vi "1DTurnMainTester.vi"() -> ()   [LabVIEW 2017]
uses:
  <vilib>/Rock Robotics/WPI/SafetyOutput/WPI_SafetyOutputConfigMenu.ctl
  <vilib>/Rock Robotics/SystemInterfaces/DIO/FPGA_DIOPWMChannel.ctl
  <vilib>/Rock Robotics/SystemInterfaces/DIO/FPGA_DIOChannel.ctl
  <extravilib>/ChannelInstances/Lossy Stream-c(dbl,dbl,dbl,dbl,dbl,dbl)/Write With Abort.vi
  <extravilib>/ChannelInstances/Lossy Stream-c(dbl,dbl,dbl,dbl,dbl,dbl)/Read With Abort.vi
  <extravilib>/ChannelInstances/Lossy Stream-c(dbl,dbl,dbl,dbl,dbl,dbl)/Endpoint.vi
  <extravilib>/ChannelInstances/Lossy Stream-c(dbl,dbl,dbl,dbl,dbl,dbl)/EndpointRead.vi
  <vilib>/Rock Robotics/WPI/RobotDrive/WPI_RobotDriveOpen4MotorWithSPARK.vi
  <vilib>/Rock Robotics/WPI/RobotDrive/WPI_RobotDriveOpen2MotorWithSPARK.vi
  <vilib>/Rock Robotics/WPI/Counter/WPI_CounterDigitalInputToDigitalSource.vi
  <extravilib>/ChannelInstances/Lossy Stream-c(dbl,dbl,dbl,dbl,dbl,dbl)/Instantiate.vi
  <extravilib>/ChannelInstances/Lossy Stream-c(dbl,dbl,dbl,dbl,dbl,dbl)/)Channel.vi
  <resource>/ChannelSupport/_ChannelSupport/WaitIfNeeded.vi
  <vilib>/Rock Robotics/WPI/ThirdParty/Sensors/navX/_Processing Loop/FRIC_navX_Internal_SPI_ProcessingLoop.vi
  <extravilib>/ChannelInstances/Lossy Stream-c(dbl,dbl,dbl,dbl,dbl,dbl).lvlib
panel:
  out "Trackwidth":dbl(graph)=25.77061221384658
  in  "AutoTurnSpeed":dbl=0.7
  in  "ThingToDo":enum16{"TestTurning", "FindTrackwidth"}(ring)
  out "Encoder Position":cluster{"Distance":dbl, "CurrentAngle":dbl}(graph)
  in  "Gains":T1={"Gains"={"FFV"=0.0061, "FFA"=0.0024, "Vel PID"={"P"=0.04, "I"=0.0, "D"=0.0}}, "Pos PID"={"P"=0.1, "I"=0.05, "D"=0.0}, "MinVoltage"=0.25, "Effective Trackwidth CW"=30.0, "Effective Trackwidth CCW"=30.0} {"Pos PID"."D" format="%.3f"; "Pos PID"."I" format="%.3f"; "Pos PID"."P" format="%.3f"}
  in  "A? or B":bool=TRUE
  in  "TargetB":dbl=170.0
  out "Voltage difference":dbl(graph)=1.0
  out "Power":dbl(graph)
  out "Done?":bool=TRUE
  out "Vel":cluster{"Output":dbl, "dx/dt":dbl}(graph)
  out "Angle":cluster{"Distance":dbl, "CurrentAngle":dbl}(graph)={"Distance"=0.0, "CurrentAngle"=-1.9899999999999807}
  in  "TargetA":dbl
  in  "MaxVel":dbl=80.0
  in  "MaxAccel":dbl=100.0
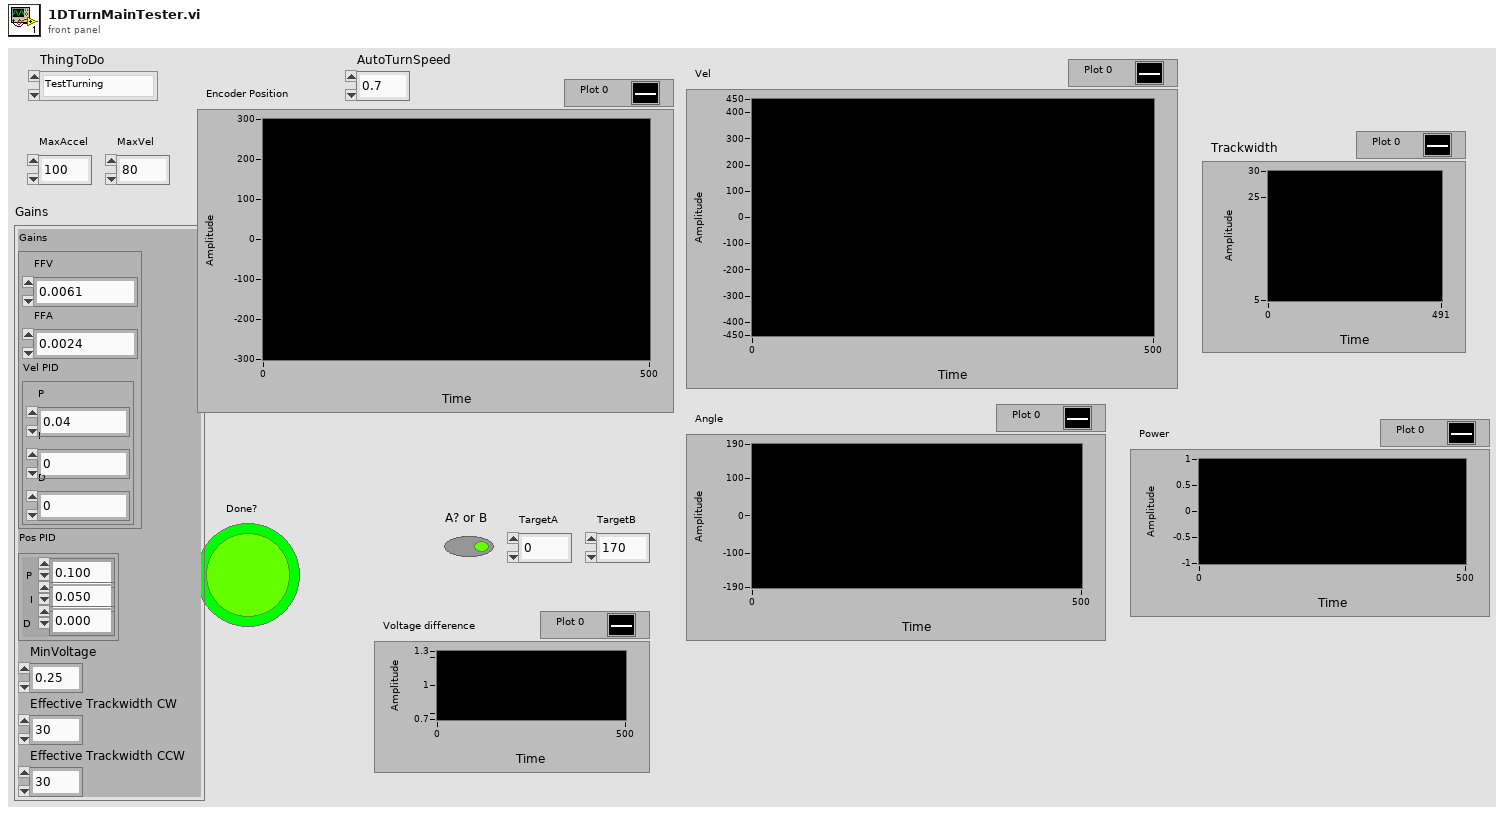
[diagram p1: front panel]
types:
  T1 = cluster{"Gains":cluster{"FFV":dbl, "FFA":dbl, "Vel PID":cluster{"P":dbl, "I":dbl, "D":dbl}}, "Pos PID":cluster{"P":dbl, "I":dbl, "D":dbl}, "MinVoltage":dbl, "Effective Trackwidth CW":dbl, "Effective Trackwidth CCW":dbl}
  T2 = typedef "FPGA_DIOChannel.ctl" = enum8{"DIO 0", "DIO 1", "DIO 2", "DIO 3", "DIO 4", "DIO 5", "DIO 6", "DIO 7", "DIO 8", "DIO 9", "DIO MXP 0", "DIO MXP 1", "DIO MXP 2", "DIO MXP 3", "DIO MXP 4", "DIO MXP 5", "DIO MXP 6", "DIO MXP 7", "DIO MXP 8", "DIO MXP 9", "DIO MXP 10", "DIO MXP 11", "DIO MXP 12", "DIO MXP 13", "DIO MXP 14", "DIO MXP 15", "SPI Port CS1", "SPI Port CS2", "SPI Port CS3", "SPI Port MISO", "SPI Port MOSI", "Invalid"}
  T3 = typedef "FPGA_DIOPWMChannel.ctl" = enum8{"PWM 0", "PWM 1", "PWM 2", "PWM 3", "PWM 4", "PWM 5", "PWM 6", "PWM 7", "PWM 8", "PWM 9", "PWM MXP 0", "PWM MXP 1", "PWM MXP 2", "PWM MXP 3", "PWM MXP 4", "PWM MXP 5", "PWM MXP 6", "PWM MXP 7", "PWM MXP 8", "PWM MXP 9", "Invalid"}
  T4 = typedef "WPI_SafetyOutputConfigMenu.ctl" = enum16{"Enable", "Disable"}
  T5 = typedef "WPI_DigitalInputDevRef.ctl" = cluster{"DevStatus":errorcluster, "DIO Channel":T2}
  T6 = typedef "FPGA_CounterEncoderSourceConvertionLVSourceType.ctl" = cluster{"DevStatus":errorcluster, "AnalogTriggerMode?":bool, "DigitalMode":cluster{"DIO Channel":T7}, "AnalogTriggerMode":cluster{"AnalogTriggerIndex":T8, "OutputType":T9}}
  T7 = typedef "FPGA_DIODigitalSourceChannel.ctl" = enum8{"DIO 0", "DIO 1", "DIO 2", "DIO 3", "DIO 4", "DIO 5", "DIO 6", "DIO 7", "DIO 8", "DIO 9", "DIO MXP 0", "DIO MXP 1", "DIO MXP 2", "DIO MXP 3", "DIO MXP 4", "DIO MXP 5", "DIO MXP 6", "DIO MXP 7", "DIO MXP 8", "DIO MXP 9", "DIO MXP 10", "DIO MXP 11", "DIO MXP 12", "DIO MXP 13", "DIO MXP 14", "DIO MXP 15", "Disabled"}
  T8 = typedef "FPGA_AnalogTriggerIndex.ctl" = enum8{"Trig 0", "Trig 1", "Trig 2", "Trig 3", "Trig 4", "Trig 5", "Trig 6", "Trig 7", "Invalid"}
  T9 = typedef "FPGA_AnalogTriggerOutType.ctl" = enum16{"InWindow", "TriggerState", "Rising", "Falling"}
  T10 = typedef "WPI_EncoderDevRef.ctl" = cluster{"DevStatus":errorcluster, "EncoderIndex":T11, "CounterIndex":T12, "DistancePerCount":dbl, "Decoding Type":T13}
  T11 = typedef "FPGA_EncoderIdx.ctl" = enum8{"Enc 0", "Enc 1", "Enc 2", "Enc 3", "Enc 4", "Enc 5", "Enc 6", "Enc 7", "Invalid"}
  T12 = typedef "FPGA_CounterCtrSystemIndex.ctl" = enum8{"Ctr 0", "Ctr 1", "Ctr 2", "Ctr 3", "Ctr 4", "Ctr 5", "Ctr 6", "Ctr 7", "Invalid"}
  T13 = typedef "WPI_EncoderType.ctl" = enum16{"1x", "2x", "4x"}
  T14 = typedef "WPI_RobotDriveDevRef.ctl" = cluster{"DevStatus":errorcluster, "Motors[]":T15[], "Square Inputs":bool, "Max Output":dbl}
  T15 = typedef "WPI_MotorControlDeviceRef.ctl" = cluster{"DeviceStatus":errorcluster, "Type":T16, "PWM":cluster{"PWM Channel":T3, "DeadBand":T17}, "CAN":cluster{"Device Number":u8, "SetOutput VI Ref":variant, "GetOutput VI Ref":variant, "Enable VI Ref":variant, "Disable VI Ref":variant, "Data":variant}, "Invert":bool, "DIO PWM":cluster{"PWM \"Enable\" Channel":T3, "DIOChannel":T2, "PWM Rate":dbl}}
  T16 = typedef "WPI_MotorControlType.ctl" = enum16{"PWM", "CAN", "DIO PWM"}
  T17 = typedef "WPI_PWMDeadband.ctl" = cluster{"Name":string, "maxPositivePwm":i32, "minPositivePwm":i32, "centerPwm":i32, "maxNegativePwm":i32, "minNegativePwm":i32, "angularRange":u16}
  T18 = cluster{"Yaw":dbl, "Roll":dbl, "Pitch":dbl, "Heading":dbl, "Fused Heading":dbl}
  T19 = cluster{dbl, "dx/dt":dbl, "Distance":dbl, "dx/dt":dbl, "Distance":dbl, "dx/dt":dbl}
  T20 = typedef "Lossy Stream-c(dbl,dbl,dbl,dbl,dbl,dbl).lvlib/)Channel.ctl" = refnum<queue>
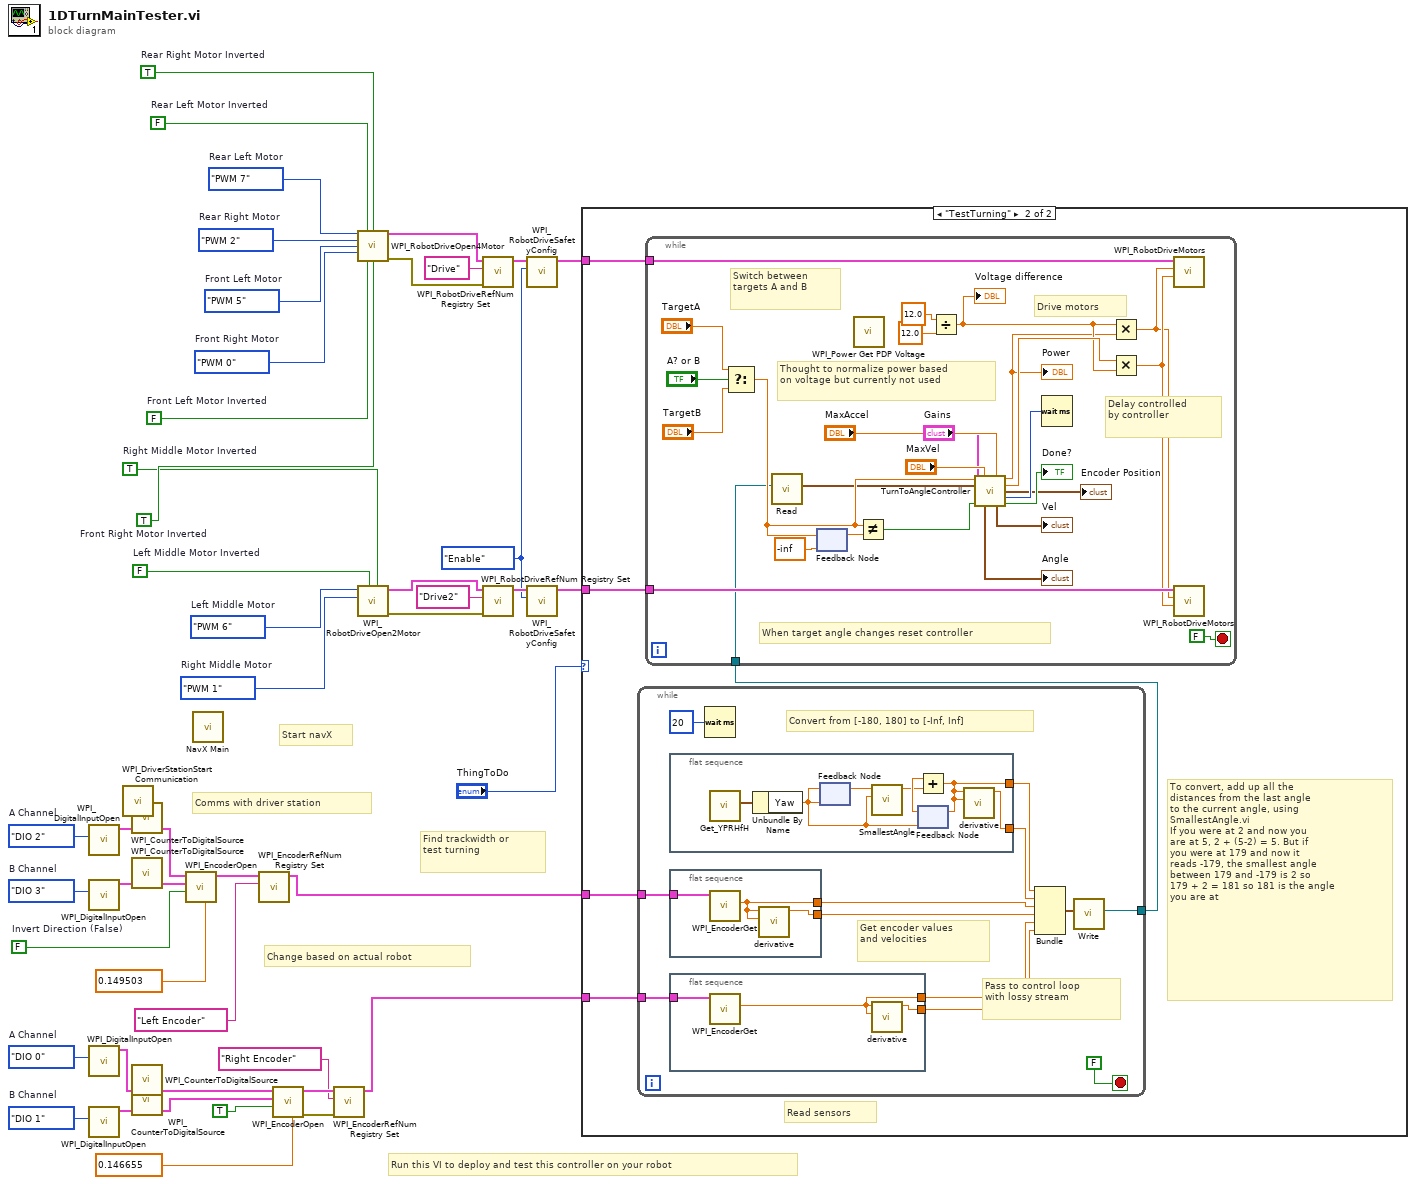
[diagram p0: block diagram]
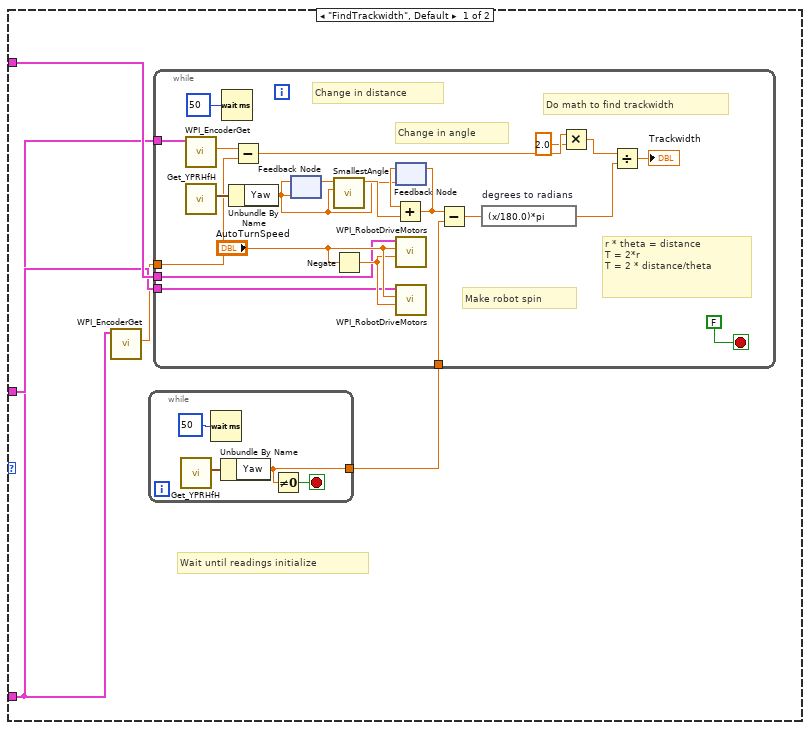
[diagram p2: hidden frame]
diagram:
  w7 = FPGA_DIOChannel."DIO 1"  # B Channel
  w10 = FPGA_DIOChannel."DIO 0"  # A Channel
  w23 = FALSE  # Invert Direction (False)
  w16 = FPGA_DIOChannel."DIO 3"  # B Channel
  w17 = FPGA_DIOChannel."DIO 2"  # A Channel
  w32 = TRUE  # Right Middle Motor Inverted
  w33 = FALSE  # Left Middle Motor Inverted
  w27 = FPGA_DIOPWMChannel."PWM 1"  # Right Middle Motor
  w36 = FPGA_DIOPWMChannel."PWM 6"  # Left Middle Motor
  w37 = TRUE  # Front Right Motor Inverted
  w38 = FALSE  # Front Left Motor Inverted
  w39 = TRUE  # Rear Right Motor Inverted
  w40 = FALSE  # Rear Left Motor Inverted
  w41 = FPGA_DIOPWMChannel."PWM 0"  # Front Right Motor
  w42 = FPGA_DIOPWMChannel."PWM 5"  # Front Left Motor
  w43 = FPGA_DIOPWMChannel."PWM 2"  # Rear Right Motor
  w44 = FPGA_DIOPWMChannel."PWM 7"  # Rear Left Motor
  w28 = WPI_SafetyOutputConfigMenu."Enable" ("mode")
  # "Change based on actual robot"
  # "Run this VI to deploy and test this controller on your robot"
  # "Find trackwidth or\ntest turning"
  # "Comms with driver station"
  # "Start navX"
  n1 = call <vilib>:"WPI_DigitalInputOpen.vi"("DIO Channel"=w17) -> ("DigitalInputDevRef"=w20:T5)  [unwired: 1 in, 9 out]
  n2 = call <vilib>:"WPI_DigitalInputOpen.vi"("DIO Channel"=w16) -> ("DigitalInputDevRef"=w19:T5)  [unwired: 1 in, 9 out]
  n3 = call <vilib>:"WPI_DigitalInputOpen.vi"("DIO Channel"=w10) -> ("DigitalInputDevRef"=w11:T5)  [unwired: 1 in, 9 out]
  n4 = call <vilib>:"WPI_DigitalInputOpen.vi"("DIO Channel"=w7) -> ("DigitalInputDevRef"=w8:T5)  [unwired: 1 in, 9 out]
  n5 = call <vilib>:"WPI_DriverStationStart Communication.vi"() -> ()  [unwired: 12 in]
  n6 = call-poly <vilib>:"WPI_CounterToDigitalSource.vi"("DigitalInputDevRef"=w20) -> ("Digital Source"=w21:T6)  [unwired: 6 out]
  n7 = call-poly <vilib>:"WPI_CounterToDigitalSource.vi"("DigitalInputDevRef"=w19) -> ("Digital Source"=w18:T6)  [unwired: 6 out]
  n8 = call-poly <vilib>:"WPI_CounterToDigitalSource.vi"("DigitalInputDevRef"=w11) -> ("Digital Source"=w12:T6)  [unwired: 6 out]
  n9 = call-poly <vilib>:"WPI_CounterToDigitalSource.vi"("DigitalInputDevRef"=w8) -> ("Digital Source"=w9:T6)  [unwired: 6 out]
  n10 = call <vilib>:"WPI_EncoderOpen.vi"("DistancePerCount"=0.149503, "Invert Direction (False)"=w23, "BSource"=w18, "ASource"=w21) -> ("EncoderDevRef"=w22:T10)  [unwired: 4 in, 3 out]
  n11 = call-poly <vilib>:"NavX Main.vi"() -> ()  [unwired: 12 in]
  n12 = call <vilib>:"WPI_EncoderRefNum Registry Set.vi"("refnum name"="Left Encoder", "EncoderDevRef"=w22) -> ("EncoderDevRef"=w3:T10)  [unwired: 8 in, 1 out]
  n13 = call <vilib>:"WPI_EncoderOpen.vi"("DistancePerCount"=0.146655, "Invert Direction (False)"=TRUE, "BSource"=w9, "ASource"=w12) -> ("error out"=w14:errorcluster, "EncoderDevRef"=w13:T10)  [unwired: 4 in, 2 out]
  n14 = call <vilib>:"WPI_EncoderRefNum Registry Set.vi"("error in (no error)"=w14, "refnum name"="Right Encoder", "EncoderDevRef"=w13) -> ("EncoderDevRef"=w2:T10)  [unwired: 7 in, 1 out]
  n15 = call-poly <vilib>:"WPI_RobotDriveOpen4Motor.vi"("Rear Left Motor"=w44, "Rear Left Motor Inverted"=w40, "Rear Right Motor Inverted"=w39, "Rear Right Motor"=w43, "Front Left Motor"=w42, "Front Right Motor"=w41, "Front Left Motor Inverted"=w38, "Front Right Motor Inverted"=w37) -> ("RobotDriveDevRef"=w47:T14, "error out"=w45:errorcluster)  [unwired: 6 in]
  n16 = call-poly <vilib>:"WPI_RobotDriveOpen2Motor.vi"("Right Motor Inverted"=w32, "Left Motor Inverted"=w33, "Right Motor"=w27, "Left Motor"=w36) -> ("error out"=w31:errorcluster, "RobotDriveDevRef"=w35:T14)  [unwired: 6 in]
  n17 = call <vilib>:"WPI_RobotDriveRefNum Registry Set.vi"("error in (no error)"=w45, "refnum name"="Drive", "RobotDriveDevRef"=w47) -> ("RobotDriveDevRef"=w30:T14)  [unwired: 1 in, 7 out]
  n18 = call <vilib>:"WPI_RobotDriveRefNum Registry Set.vi"("error in (no error)"=w31, "refnum name"="Drive2", "RobotDriveDevRef"=w35) -> ("RobotDriveDevRef"=w29:T14)  [unwired: 7 in, 1 out]
  n19 = call <vilib>:"WPI_RobotDriveSafetyConfig.vi"("mode"=w28, "RobotDriveDevRef"=w30) -> ("RobotDriveDevRef"=w25:T14)  [unwired: 8 in, 1 out]
  n20 = call <vilib>:"WPI_RobotDriveSafetyConfig.vi"("mode"=w28, "RobotDriveDevRef"=w29) -> ("RobotDriveDevRef"=w26:T14)  [unwired: 8 in, 1 out]
  n21 = case shown="\"TestTurning\"" "ThingToDo" {
    tunnel: w26 -> [w51 w83]
    tunnel: w25 -> [w52 w82]
    tunnel: w3 -> [w50 w81]
    tunnel: w2 -> [_ w80]
    frame "FindTrackwidth", Default {
      # "Wait until readings initialize"
      n22 = call <vilib>:"WPI_EncoderGet.vi"("EncoderDevRef"=w50) -> ("Distance"=w49:dbl)  [unwired: 5 in, 5 out]
      n23 = while {
        tunnel: [w53] -> w48
        stop <- w55 stop-if-true
        n24 = call <vilib>:"Get_YPRHfH.vi"() -> ("YRPHfH"=w56:T18)  [unwired: 11 in]
        n25 = Wait (ms)(milliseconds to wait=u32 50) -> ()  [unwired: 1 out]
        n26 = Unbundle By Name(w56) -> ("Yaw"=w53:dbl)
        n27 = Not Equal To 0?(x=w53) -> (x != 0?=w55:bool)
      }
      n28 = while {
        tunnel: w52 -> [w74]
        tunnel: w51 -> [w73]
        tunnel: w50 -> [w68]
        tunnel: w49 -> [w66]
        tunnel: w48 -> [w60]
        stop <- FALSE stop-if-true
        # "r * theta = distance\nT = 2*r\nT = 2 * distance/theta"
        # "Do math to find trackwidth"
        # "Make robot spin"
        # "Change in angle"
        # "Change in distance"
        n29 = call <vilib>:"WPI_EncoderGet.vi"("EncoderDevRef"=w68) -> ("Distance"=w67:dbl)  [unwired: 5 in, 5 out]
        n30 = call <vilib>:"Get_YPRHfH.vi"() -> ("YRPHfH"=w72:T18)  [unwired: 11 in]
        n31 = Wait (ms)(milliseconds to wait=u32 50) -> ()  [unwired: 1 out]
        n32 = Unbundle By Name(w72) -> ("Yaw"=w61:dbl)
        n33 = Subtract(x=w67, y=w66) -> (x-y=w59:dbl)
        n34 = feedback #1(w61) -> (w69:dbl)
        n35 = feedback-in #1(w61) -> ()
        n36 = call "SmallestAngle.vi"("Angle B"=w61, "Angle A"=w69) -> ("Smallest A to B"=w70:dbl)  [unwired: 9 in]
        n37 = Negate(x="AutoTurnSpeed") -> (-x=w77:dbl)
        n38 = feedback #2(w61) -> (w71:dbl)
        n39 = Add(x=w71, y=w70) -> (x+y=w65:dbl)
        n40 = feedback-in #2(w65) -> ()
        n41 = call <vilib>:"WPI_RobotDriveMotors.vi"("RightSpeed"=w77, "LeftSpeed"="AutoTurnSpeed", "RobotDriveDevRef"=w74) -> ()  [unwired: 1 in, 8 out]
        n42 = call <vilib>:"WPI_RobotDriveMotors.vi"("RightSpeed"=w77, "LeftSpeed"="AutoTurnSpeed", "RobotDriveDevRef"=w73) -> ()  [unwired: 1 in, 8 out]
        n43 = Subtract(x=w65, y=w60) -> (x-y=w64:dbl)
        n44 = expression code="(x/180.0)*pi" "degrees to radians"(w64) -> (w63:dbl)
        n45 = Multiply(x=w59, y=2.0) -> (x*y=w57:dbl)
        n46 = Divide(x=w57, y=w63) -> (x/y=→"Trackwidth":dbl)
      }
    }
    frame "TestTurning" {
      # "To convert, add up all the\ndistances from the last angle\nto the current angle, using\nSmallestAngle.vi\nIf you were at 2 and now you\nare at 5, 2 + (5-2) = 5. But if\nyou were at 179 and now it\nreads -179, the smallest angle\nbetween 179 and -179 is 2 so\n179 + 2 = 181 so 181 is the angle\nyou are at"
      # "Read sensors"
      n47 = while {
        tunnel: w81 -> [w91]
        tunnel: w80 -> [w90]
        tunnel: [w84] -> w79
        stop <- FALSE stop-if-true
        # "Pass to control loop\nwith lossy stream"
        # "Get encoder values\nand velocities"
        # "Convert from [-180, 180] to [-Inf, Inf]"
        n48 = flat-sequence {
          tunnel: [w107] -> w92
          tunnel: [w103] -> w93
          frame #0 {
            n49 = call <vilib>:"Get_YPRHfH.vi"() -> ("YRPHfH"=w108:T18)  [unwired: 11 in]
            n50 = Unbundle By Name(w108) -> ("Yaw"=w102:dbl)
            n51 = feedback #3(w102) -> (w104:dbl)
            n52 = feedback-in #3(w102) -> ()
            n53 = call "SmallestAngle.vi"("Angle B"=w102, "Angle A"=w104) -> ("Smallest A to B"=w105:dbl)  [unwired: 9 in]
            n54 = feedback #4(w102) -> (w106:dbl)
            n55 = Add(x=w106, y=w105) -> (x+y=w103:dbl)
            n56 = feedback-in #4(w103) -> ()
            n57 = call "derivative.vi"("Starting value"=w103, "x"=w103) -> ("dx/dt"=w107:dbl)  [unwired: 9 in]
          }
        }
        n58 = flat-sequence {
          tunnel: [w98] -> w88
          tunnel: [w97] -> w89
          tunnel: w91 -> [w96]
          frame #0 {
            n59 = call <vilib>:"WPI_EncoderGet.vi"("EncoderDevRef"=w96) -> ("Distance"=w97:dbl)  [unwired: 5 in, 5 out]
            n60 = call "derivative.vi"("Starting value"=w97, "x"=w97) -> ("dx/dt"=w98:dbl)  [unwired: 9 in]
          }
        }
        n61 = flat-sequence {
          tunnel: [w100] -> w86
          tunnel: [w99] -> w87
          tunnel: w90 -> [w101]
          frame #0 {
            n62 = call <vilib>:"WPI_EncoderGet.vi"("EncoderDevRef"=w101) -> ("Distance"=w99:dbl)  [unwired: 5 in, 5 out]
            n63 = call "derivative.vi"("Starting value"=w99, "x"=w99) -> ("dx/dt"=w100:dbl)  [unwired: 9 in]
          }
        }
        n64 = Wait (ms)(milliseconds to wait=u32 20) -> ()  [unwired: 1 out]
        n65 = Bundle(w93, "dx/dt"=w92, "Distance"=w89, "dx/dt"=w88, "Distance"=w87, "dx/dt"=w86) -> (w85:T19)  [unwired: 1 in]
        n66 = call <extravilib>:"Write.vi"("element"=w85) -> ("channel"=w84:T20)  [unwired: 8 in, 2 out]
      }
      n67 = while {
        tunnel: w83 -> [w126]
        tunnel: w82 -> [w125]
        tunnel: w79 -> [w113]
        stop <- FALSE stop-if-true
        # "Delay controlled\nby controller"
        # "Thought to normalize power based\non voltage but currently not used"
        # "Drive motors"
        # "When target angle changes reset controller"
        # "Switch between\ntargets A and B"
        n68 = Select(t="TargetA", s="A? or B", f="TargetB") -> (s? t:f=w114:dbl)
        n69 = call <extravilib>:"Read.vi"("channel"=w113) -> ("element"=w112:T19)  [unwired: 5 in, 5 out]
        n70 = feedback-in #5(w114) -> ()
        n71 = feedback #5(-inf ("TargetAngle")) -> (w128:dbl)
        n72 = call <vilib>:"WPI_Power Get PDP Voltage.vi"() -> ()  [unwired: 14 in, 2 out]
        n73 = Not Equal?(x=w114, y=w128) -> (x != y?=w127:bool)
        n74 = Divide(x=12.0, y=12.0) -> (x/y=w120:dbl)
        "Voltage difference" <- w120
        n75 = call "TurnToAngleController.vi"("TargetAngle"=w114, "MaxVel"="MaxVel", "MaxAccel"="MaxAccel", "Robot"=w112, "Gains"="Gains", "Reset"=w127) -> ("LeftPower"=w110:dbl, "RightPower"=w122:dbl, "Encoder Distance"=→"Encoder Position":cluster{"Output":dbl, "dx/dt":dbl}, "Delay"=w134:u32, "Angle"=→"Angle":cluster{"Distance":dbl, "CurrentAngle":dbl}, "VelGraph"=→"Vel":cluster{"Output":dbl, "dx/dt":dbl}, "Done"=→"Done?":bool)  [unwired: 3 in]
        "Power" <- w110
        n76 = Wait (ms)(milliseconds to wait=w134) -> ()  [unwired: 1 out]
        n77 = Multiply(x=w120, y=w110) -> (x*y=w119:dbl)
        n78 = Multiply(x=w122, y=w120) -> (x*y=w121:dbl)
        n79 = call <vilib>:"WPI_RobotDriveMotors.vi"("RightSpeed"=w121, "LeftSpeed"=w119, "RobotDriveDevRef"=w125) -> ()  [unwired: 1 in, 8 out]
        n80 = call <vilib>:"WPI_RobotDriveMotors.vi"("RightSpeed"=w121, "LeftSpeed"=w119, "RobotDriveDevRef"=w126) -> ()  [unwired: 1 in, 8 out]
      }
    }
  }
